vi "Wait for Connection.vi"(8 "error in (no error)":errorcluster, 9 "timeout ms (5000)":i32=5000, 11 "TinyTCP":T1) -> (0 "error out":errorcluster)   [LabVIEW 2020, in "TinyTCP.lvlib"]
doc: "Waits up to the specified timeout for the connection to be established. If this times out or there is an error the connection does not stop trying to connect until <b>Close</b> or <b>Stop</b> is called."
uses:
  TinyTCP.lvlib
  State.ctl
  Ref Data.ctl
  Instance.ctl
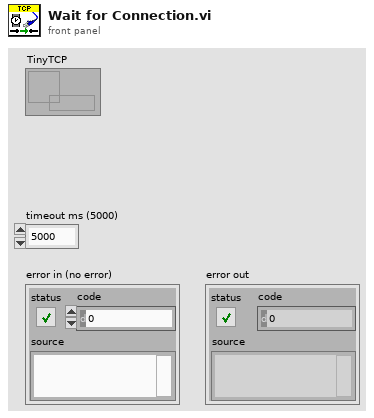
[diagram p1: front panel]
types:
  T1 = typedef "TinyTCP.lvlib/Instance.ctl" = refnum<data-value>
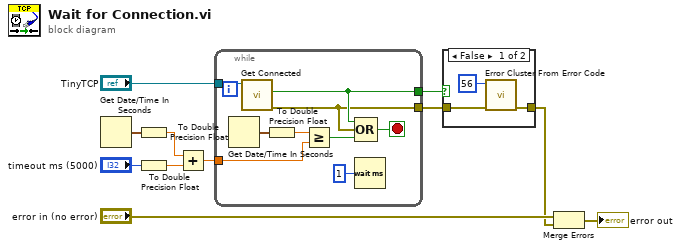
[diagram p0: block diagram]
diagram:
  n1 = Get Date/Time In Seconds() -> (seconds since 1Jan1904=w10:timestamp)
  n2 = To Double Precision Float(number=w10) -> (double precision float=w9:dbl)
  n3 = To Double Precision Float(number="timeout ms (5000)") -> (double precision float=w8:dbl)
  n4 = Add(x=w9, y=w8) -> (x+y=w7:dbl)
  n5 = while {
    tunnel: w7 -> [w17]
    tunnel: "TinyTCP" -> [w20]
    tunnel: [w16] -> w5
    tunnel: [w12] -> w4
    stop <- w14 stop-if-true
    n6 = Get Date/Time In Seconds() -> (seconds since 1Jan1904=w19:timestamp)
    n7 = call "Get Connected.vi"("TCP Comm"=w20) -> ("error out"=w12:errorcluster, "Connected"=w16:bool)  [unwired: 9 in]
    n8 = To Double Precision Float(number=w19) -> (double precision float=w18:dbl)
    n9 = Greater Or Equal?(x=w18, y=w17) -> (x >= y?=w15:bool)
    n10 = Compound Arithmetic op=OR(w16, w12, w15) -> (w14:bool)
    n11 = Wait (ms)(milliseconds to wait=u32 1) -> ()  [unwired: 1 out]
  }
  n12 = case shown="False" w5 {
    tunnel: w4 -> [w23 w24]
    tunnel: [w21 w24] -> w2
    frame False {
      n13 = call <vilib>:"Error Cluster From Error Code.vi"("error in (no error)"=w23, "error code (0)"=56) -> ("error out"=w21:errorcluster)  [unwired: 7 in]
    }
    frame True {
    }
  }
  n14 = Merge Errors("error in (no error)", w2) -> (→"error out":errorcluster)
